vi "Write User Attributes.vi"(8 "error in (no error)":errorcluster, 10 "User attributes":T1={"Observer"="ECHARPE", "Object"="UNDEFINED", "Program ID"="UNDEFINED", "Night Directory"=""}, 11 "User in":refnum<class "User.lvclass">) -> (0 "error out":errorcluster, 3 "User out":refnum<class "User.lvclass">)   [LabVIEW 2018, in "User.lvclass"]
doc: "Este VI escreve na classe os valores de cada atributo do usuário."
uses:
  User.lvclass
  User.lvclass/User.ctl
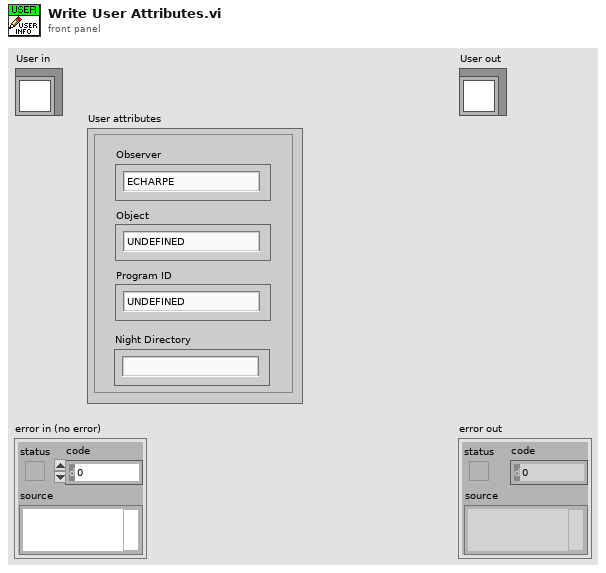
[diagram p1: front panel]
types:
  T1 = cluster{"Observer":string, "Object":string, "Program ID":string, "Night Directory":string}
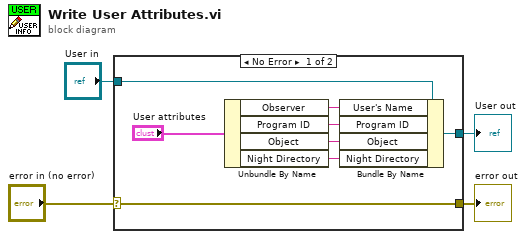
[diagram p0: block diagram]
diagram:
  n1 = case shown="No Error" "error in (no error)" {
    selector: "error in (no error)" -> [w12 w14]
    tunnel: [w12 w14] -> w3
    tunnel: [w10 w13] -> w1
    tunnel: "User in" -> [w11 w13]
    frame No Error {
      n2 = Unbundle By Name("User attributes") -> ("Observer"=w5:string, "Program ID"=w6:string, "Object"=w7:string, "Night Directory"=w8:string)
      n3 = Bundle By Name(cluster=w11, "User's Name"=w5, "Program ID"=w6, "Object"=w7, "Night Directory"=w8) -> (w10:refnum<class "User.lvclass">)
    }
    frame Error {
    }
  }
  "error out" <- w3
  "User out" <- w1
